vi "printStatus.vi"(8 "error in (no error)":errorcluster, 11 "Radio in":refnum<class "Radio.lvclass">) -> (0 "error out":errorcluster, 3 "Radio out":refnum<class "Radio.lvclass">)   [LabVIEW 2017, in "Radio.lvclass"]
uses:
  Radio.lvclass
  Radio.lvclass/Radio.ctl
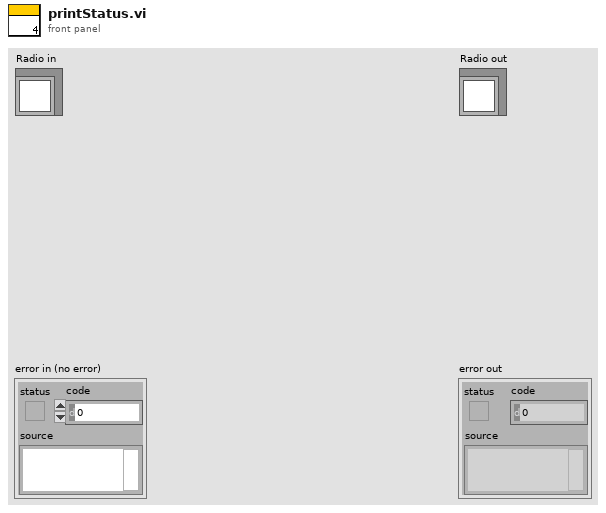
[diagram p1: front panel]
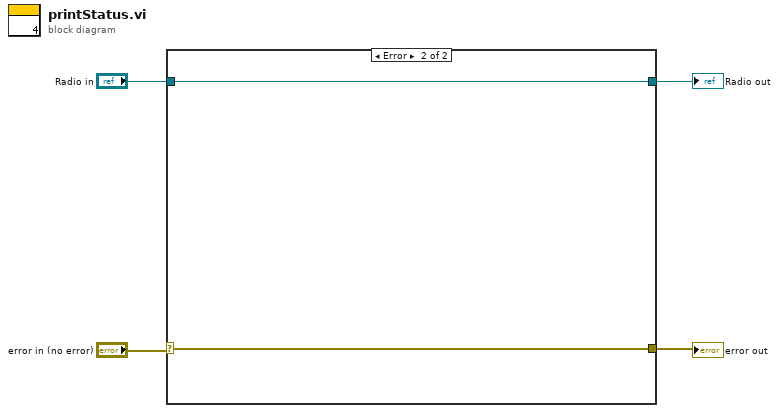
[diagram p0: block diagram]
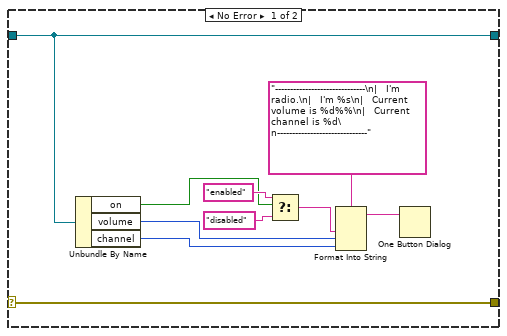
[diagram p2: hidden frame]
diagram:
  n1 = case shown="Error" "error in (no error)" {
    selector: "error in (no error)" -> [w5 w15]
    tunnel: "Radio in" -> [w6 w16]
    tunnel: [w6 w16] -> w3
    tunnel: [w5 w15] -> w1
    frame No Error {
      n2 = Unbundle By Name(w6) -> ("on"=w11:bool, "volume"=w9:i32, "channel"=w8:i32)
      n3 = Select(t="enabled", s=w11, f="disabled") -> (s? t:f=w10:string)
      n4 = Format Into String(format string="------------------------------\n|   I'm radio.\n|   I'm %s\n|   Current volume is %d%%\n|   Current channel is %d\n------------------------------", w10, w9, w8) -> (resulting string=w7:string)  [unwired: 2 in, 1 out]
      n5 = One Button Dialog(message=w7) -> ()  [unwired: 1 in, 1 out]
    }
    frame Error {
    }
  }
  "error out" <- w1
  "Radio out" <- w3
